vi "FRCts20_WebMethods_ReadData_Request.vi"(8 "error in (no error)":errorcluster, 10 "Request":T1, 11 "httpRequestID":u32) -> (0 "error out":errorcluster, 2 "Request 2":T1, 3 "httpRequestID out":u32)   [LabVIEW 2014, in "FRCts20_WebMethods.lvlib"]
uses:
  FRCts20_WebMethods.lvlib
  <vilib>/wsapi/NI_WebServices.lvlib
  Backend/source/VI Source/FRCts20_Backend_API/FRCts20_Backend_API_Status.ctl
  Backend/source/VI Source/FRCts20_Backend_API/FRCts20_Backend_API.lvlib
  Web Method Public Interface/FRCts20_WebMethods_ctl_request.ctl
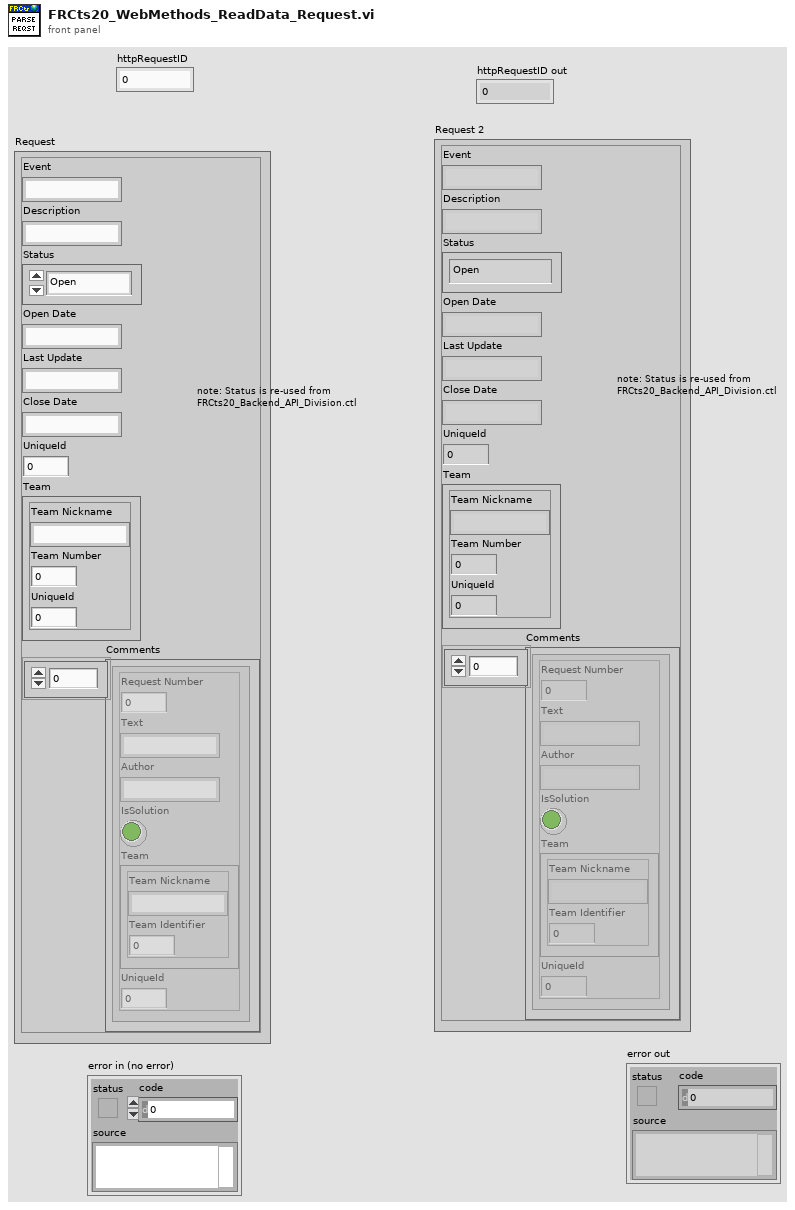
[diagram p1: front panel]
types:
  T1 = typedef "FRCts20_WebMethods.lvlib/FRCts20_WebMethods_ctl_request.ctl" = cluster{"Event":string, "Description":string, "Status":T2, "Open Date":string, "Last Update":string, "Close Date":string, "UniqueId":i32, "Team":cluster{"Team Nickname":string, "Team Number ":i32, "UniqueId":i32}, "Comments":cluster{"Request Number":dbl, "Text":string, "Author":string, "IsSolution":bool, "Team":cluster{"Team Nickname":string, "Team Identifier ":dbl}, "UniqueId":i32}[]}
  T2 = typedef "FRCts20_Backend_API.lvlib/FRCts20_Backend_API_Status.ctl" = enum16{"Open", "In Work", "Closed"}
  T3 = typedef "FRCts20_WebMethods.lvlib/FRCts20_WebMethods_ctl_returntype.ctl" = string
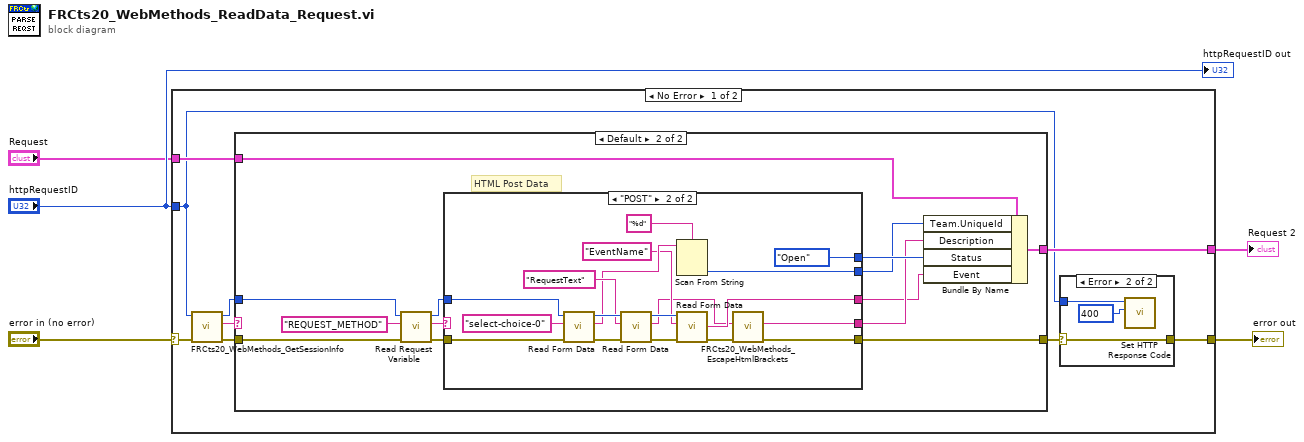
[diagram p0: block diagram]
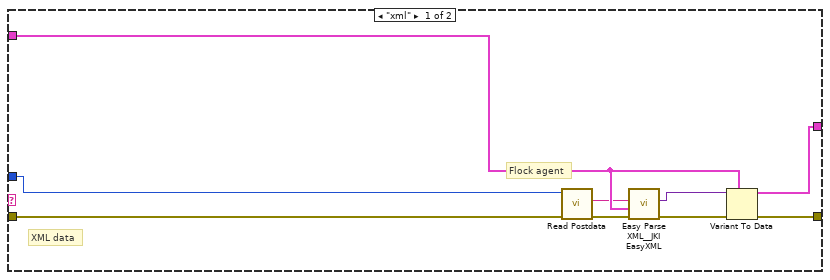
[diagram p3: hidden frame]
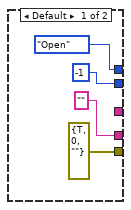
[diagram p4: hidden frame]
diagram:
  n1 = case shown="No Error" "error in (no error)" {
    selector: "error in (no error)" -> [w9 w64]
    tunnel: "httpRequestID" -> [w8 _]
    tunnel: "Request" -> [w14 w63]
    tunnel: [w11 w64] -> w4
    tunnel: [w12 w63] -> w1
    frame No Error {
      n2 = call "FRCts20_WebMethods_GetSessionInfo.vi"("error in"=w9, "httpRequestID"=w8) -> ("error out"=w10:errorcluster, "Return Type"=w7:T3, "httpRequestID out"=w6:u32)  [unwired: 7 in]
      n3 = case shown="Default" w7 {
        tunnel: w10 -> [w22 w36]
        tunnel: w14 -> [w25 w39]
        tunnel: [w24 w40] -> w13
        tunnel: [w23 w38] -> w12
        tunnel: w6 -> [w19 w29]
        frame "xml" {
          # "Flock agent"
          # "XML data"
          n4 = call <vilib>:"Read Postdata.vi"("error in (no error)"=w22, "httpRequestID"=w19) -> ("error out"=w21:errorcluster, "postdata"=w20:string)  [unwired: 7 in, 1 out]
          n5 = call <vilib>:"Easy Parse XML__JKI EasyXML.vi"("error in (no error)"=w21, "LabVIEW Data (Type)"=w25, "XML String"=w20) -> ("error out"=w27:errorcluster, "LabVIEW Data"=w26:variant)  [unwired: 7 in]
          n6 = Variant To Data(error in=w27, type=w25, Variant=w26) -> (data=w23:T1, error out=w24:errorcluster)
        }
        frame Default {
          # "HTML Post Data"
          n7 = call <vilib>:"Read Request Variable.vi"("error in (no error)"=w36, "variable name"="REQUEST_METHOD", "httpRequestID"=w29) -> ("error out"=w35:errorcluster, "value"=w34:string, "httpRequestID out"=w33:u32)  [unwired: 6 in]
          n8 = case shown="\"POST\"" w34 {
            tunnel: [errorcluster {"status"=TRUE, "code"=0, "source"=""} ("error out") w45] -> w40
            tunnel: ["" ("value") w47] -> w31
            tunnel: [-1 w54] -> w30
            tunnel: [FRCts20_Backend_API_Status."Open" ("Status") FRCts20_Backend_API_Status."Open" ("Status")] -> w32
            tunnel: w35 -> [_ w59]
            tunnel: w33 -> [_ w58]
            tunnel: [_ w49] -> w28
            frame Default {
            }
            frame "POST" {
              n9 = call <vilib>:"Read Form Data.vi"("error in (no error)"=w59, "key"="select-choice-0", "httpRequestID"=w58) -> ("error out"=w60:errorcluster, "value"=w55:string, "httpRequestID out"=w61:u32)  [unwired: 5 in, 1 out]
              n10 = call <vilib>:"Read Form Data.vi"("error in (no error)"=w60, "key"="RequestText", "httpRequestID"=w61) -> ("error out"=w51:errorcluster, "value"=w48:string, "httpRequestID out"=w52:u32)  [unwired: 5 in, 1 out]
              n11 = Scan From String(format string="%d", input string=w55) -> (output 1=w54:i32)  [unwired: 3 in, 3 out]
              n12 = call <vilib>:"Read Form Data.vi"("error in (no error)"=w51, "key"="EventName", "httpRequestID"=w52) -> ("error out"=w46:errorcluster, "value"=w49:string)  [unwired: 5 in, 2 out]
              n13 = call "FRCts20_WebMethods_EscapeHtmlBrackets.vi"("error in (no error)"=w46, "HTML String In"=w48) -> ("error out"=w45:errorcluster, "result string"=w47:string)  [unwired: 8 in]
            }
          }
          n14 = Bundle By Name(cluster=w39, "Team.UniqueId"=w30, "Description"=w31, "Status"=w32, "Event"=w28) -> (w38:T1)
        }
      }
      n15 = case shown="Error" w13 {
        selector: w13 -> [w15 w16]
        tunnel: [w15 w16] -> w11
        tunnel: w8 -> [_ w17]
        frame No Error {
        }
        frame Error {
          w18 = 400 items=["100"=100, "101"=101, "200"=200, "201"=201, "202"=202, "203"=203, "204"=204, "205"=205, "206"=206, "300"=300, "301"=301, "302"=302, "303"=303, "304"=304, "305"=305, "306"=306, "307"=307, "400"=400, "401"=401, "402"=402, "403"=403, "404"=404, "405"=405, "406"=406, "407"=407, "408"=408, "409"=409, "410"=410, "411"=411, "412"=412, "413"=413, "414"=414, "415"=415, "416"=416, "417"=417, "500"=500, "501"=501, "502"=502, "503"=503, "504"=504, "505"=505] ("response code (200)")
          n16 = call <vilib>:"Set HTTP Response Code.vi"("response code (200)"=w18, "httpRequestID"=w17) -> ()  [unwired: 8 in, 2 out]
        }
      }
    }
    frame Error {
    }
  }
  "Request 2" <- w1
  "error out" <- w4
  "httpRequestID out" <- "httpRequestID"
